vi "SubVI of the Github Demo.vi"(8 "error in (no error)":errorcluster) -> (3 "x+y":dbl)   [LabVIEW 2016]
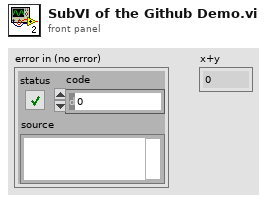
[diagram p1: front panel]
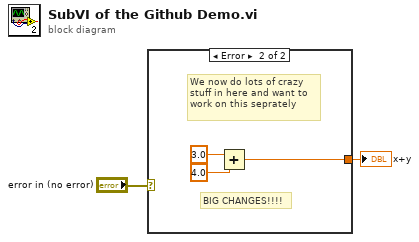
[diagram p0: block diagram]
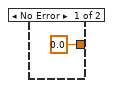
[diagram p2: hidden frame]
diagram:
  n1 = case shown="Error" "error in (no error)" {
    tunnel: [0.0 w4] -> w2
    frame No Error {
    }
    frame Error {
      # "BIG CHANGES!!!!"
      # "We now do lots of crazy\nstuff in here and want to\nwork on this seprately"
      n2 = Add(x=3.0, y=4.0) -> (x+y=w4:dbl)
    }
  }
  "x+y" <- w2
